vi "Map to Array of Clusters.vi"(8 "error in":errorcluster, 11 "Map":variant) -> (0 "error out":errorcluster, 3 "Array of Clusters (key-value)":variant)   [LabVIEW 2024, in "JSONtext.lvlib" / "SetMap.lvlib"]
uses:
  SetMap.lvlib
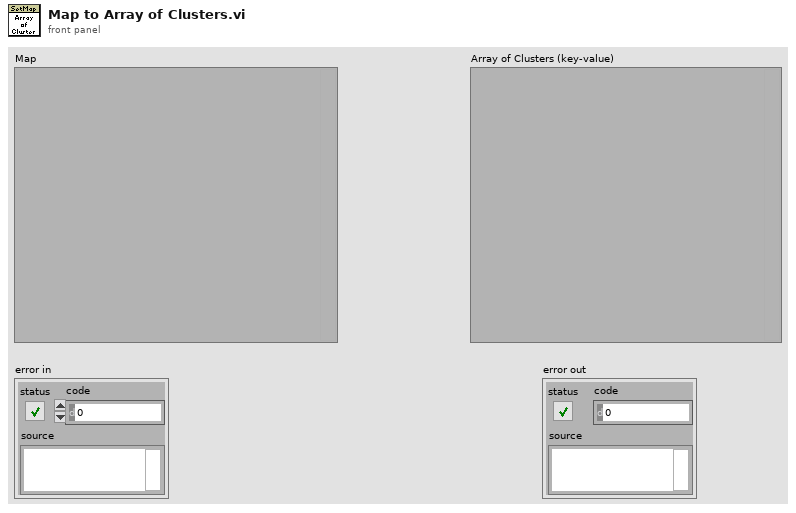
[diagram p1: front panel]
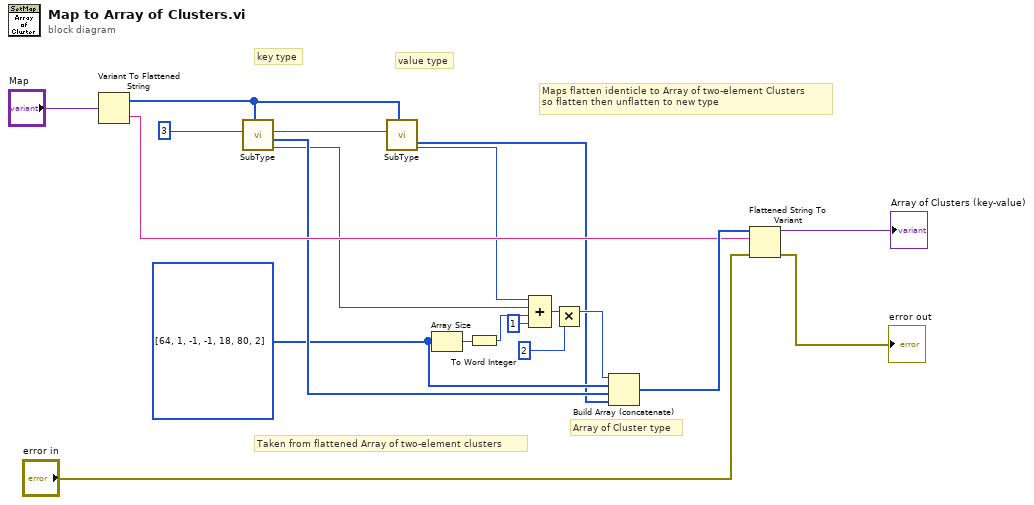
[diagram p0: block diagram]
diagram:
  w11 = i16[] [64, 1, -1, -1, 18, 80, 2] ("type string 7")
  # "Taken from flattened Array of two-element clusters"
  # "Maps flatten identicle to Array of two-element Clusters\nso flatten then unflatten to new type"
  # "value type"
  # "key type"
  # "Array of Cluster type"
  n1 = Variant To Flattened String(Variant="Map") -> (data string=w13:string, 1:w3:i16[])
  n2 = call "SubType.vi"("type"=w3, "Offset In"=i16 3 ("index")) -> ("Size"=w5:i16, "subtype"=w12:i16[], "Offset out"=w4:i16)  [unwired: 7 in]
  n3 = call "SubType.vi"("type"=w3, "Offset In"=w4) -> ("Size"=w1:i16, "subtype"=w2:i16[])  [unwired: 7 in, 1 out]
  n4 = Array Size(array=w11) -> (size(s)=w10:i32)
  n5 = To Word Integer(number=w10) -> (16bit integer=w8:i16)
  n6 = Compound Arithmetic op=ADD(w1, w5, w8, i16 1 ("value")) -> (w9:i16)
  n7 = Multiply(x=w9, y=i16 2) -> (x*y=w15:i16)
  n8 = Build Array (concatenate)(w15, w11, w12, w2) -> (w14:i16[])
  n9 = Flattened String To Variant(4:"error in", 6:w13, 7:w14) -> (0:→"error out":errorcluster, 3:→"Array of Clusters (key-value)":variant)
